vi "Sweep Pattern Dialog.vi"(8 "error in (no error)":errorcluster, 11 "Sweep Settings In":T1 {"Sweep Max" format="%#_6p"; "Sweep Min" format="%#_6p"; "Sweep Type" items=["Single Point", "Sweep", "List"]}) -> (0 "error out":errorcluster, 1 "Cancelled?":bool, 2 "Values":dbl[](array[numeric]), 3 "Sweep Settings Out":T1={"Sweep Type"=0, "Quantity"=enum."Undefined", "Base Unit"=enum."No", "Convention Unit"=enum."No", "Sweep Min"=0.0, "Sweep Max"=0.0, "Sweep NrOfPts"=0, "Values"=[0.0]} {"Sweep Max" format="%#_6p"; "Sweep Min" format="%#_6p"; "Sweep Type" items=["Single Point", "Sweep", "List"]})   [LabVIEW 2023, in "NI_HFNetworkAnalysis.lvlib"]
doc: "Dialog box allowing one to define a sweep pattern for double-precision floating point values."
uses:
  NI_HFNetworkAnalysis.lvlib
  Controls/SweepSettings.ctl
  Controls/Quantity.ctl
  Controls/Unit.ctl
  <vilib>/Utility/miscctls.llb/LVRowAndColumnTypeDef.ctl
  Support VIs/Convert Unit (DBL).vi
  Support VIs/Convert Unit (DBL Array).vi
panel:
  in  "Panel":enum32{"Page 1", "Page 3"}(tab)
  in  "Sweep Settings":T4 caption="Single" {"value3" format="%#_6p"; "value2" format="%#_6p"; "value1" format="%#_6p"}
  in  "Custom Value":T5 {"value1" format="%#_6p"}
  out "Custom List":string[][](table)
  in  "Cancel Button":bool
  in  "OK Button":bool
  in  "Type":u16(ring) caption="Type:" items=["Single Point", "Sweep", "List"]
  in  "Unit":u16(ring) caption="Unit:" items=["No"=0, "dB"=7]
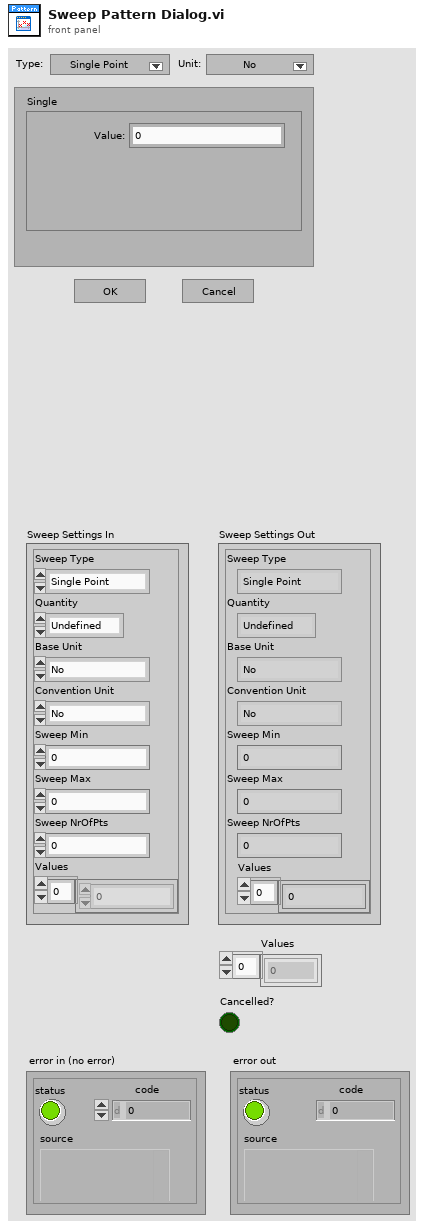
[diagram p1: front panel]
types:
  T1 = typedef "NI_HFNetworkAnalysis.lvlib/SweepSettings.ctl" = cluster{"Sweep Type":u16, "Quantity":T2, "Base Unit":T3, "Convention Unit":T3, "Sweep Min":dbl, "Sweep Max":dbl, "Sweep NrOfPts":u32, "Values":dbl[]}
  T2 = typedef "NI_HFNetworkAnalysis.lvlib/Quantity.ctl" = enum16{"Undefined", "V", "I", "A", "B", "P", "Z", "PowerRatio", "Gamma", "Index"}
  T3 = typedef "NI_HFNetworkAnalysis.lvlib/Unit.ctl" = enum16{"No", "s", "Hz", "V", "A", "Ohm", "W", "dB", "dBV", "dBA", "dBm", "percent", "rad", "deg"}
  T4 = cluster{"value1":dbl, "value2":dbl, "value3":dbl, "value4":u32, "MinMax":bool, "MinStep":bool}
  T5 = cluster{"value1":dbl, "Delete Point":bool, "Add Point":bool}
  T6 = typedef "LVRowAndColumnTypeDef.ctl" = cluster{"Row":i32, "Column":i32}
  T7 = enum8{"Enabled", "Disabled", "Disabled and Grayed Out"}
  T8 = cluster{"Sweep Type":u16, "Quantity":T2, "Base Unit":T3, "Convention Unit":u16, "Sweep Min":dbl, "Sweep Max":dbl, "Sweep NrOfPts":u32, "Values":dbl[]}
  T9 = cluster{"Sweep Type":u16, "Quantity":T2, "Base Unit":T3, "Convention Unit":u16, "regularSweepMin":dbl, "regularSweepMax":dbl, "regularSweepNrOfPts":u32, "Values":dbl[]}
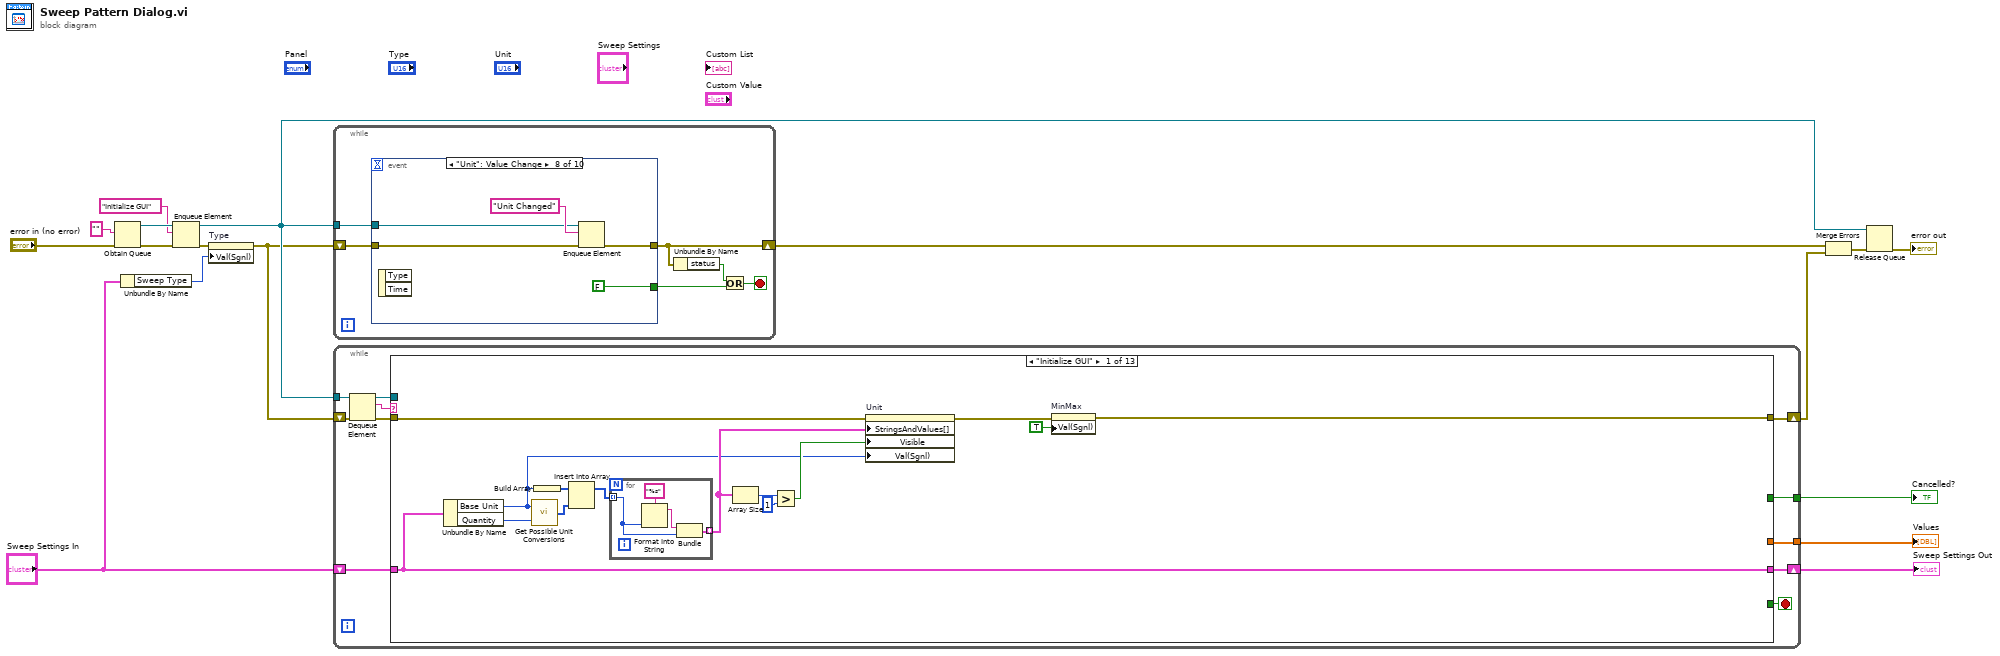
[diagram p0: block diagram]
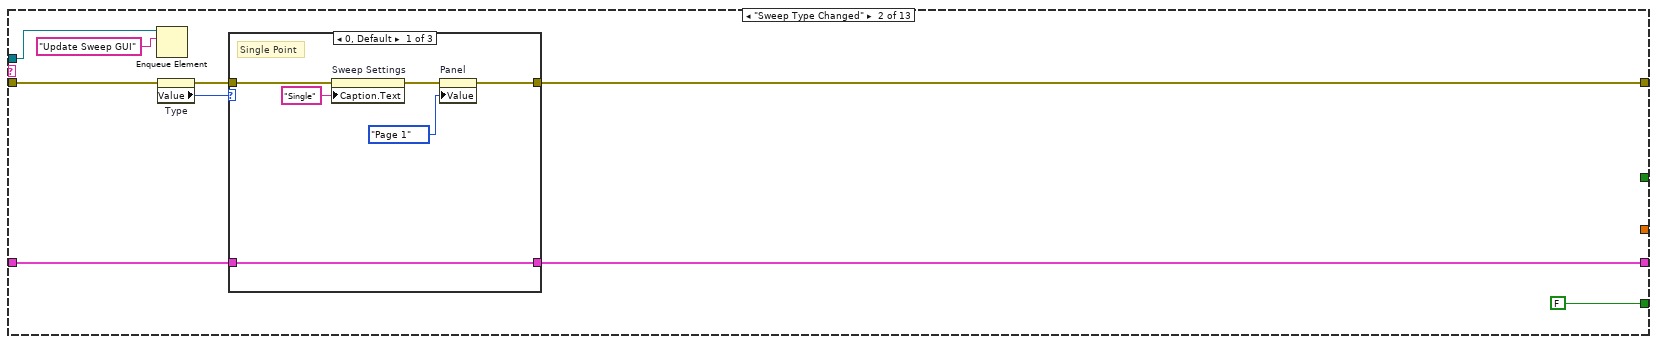
[diagram p2: hidden frame]
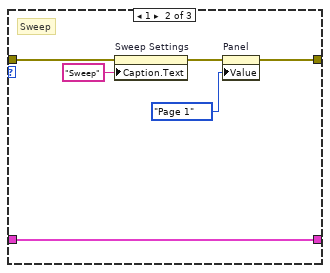
[diagram p3: hidden frame]
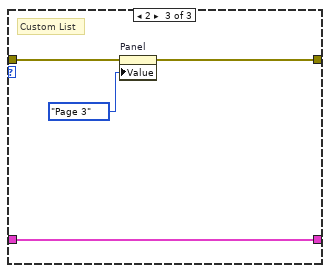
[diagram p4: hidden frame]
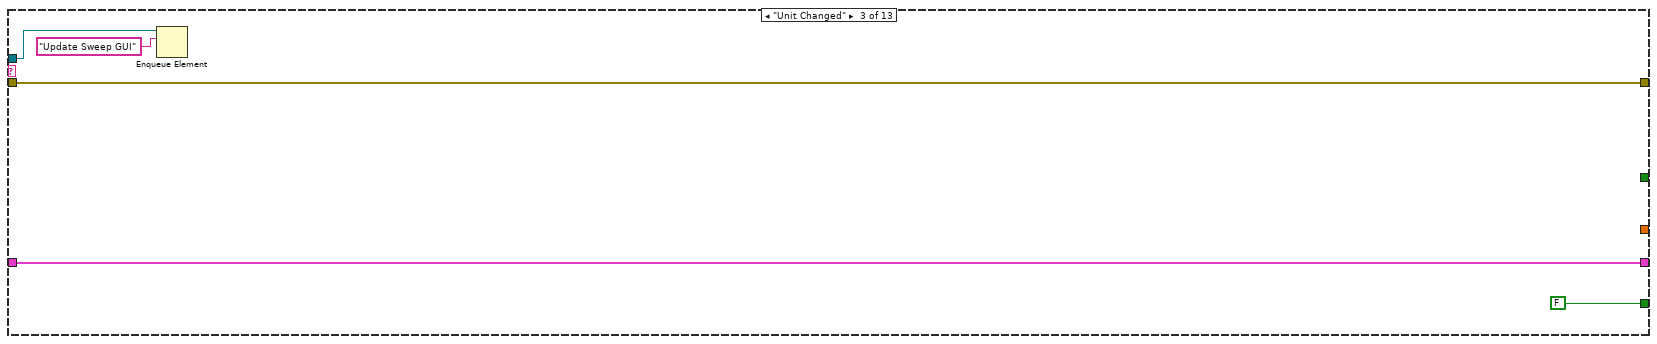
[diagram p5: hidden frame]
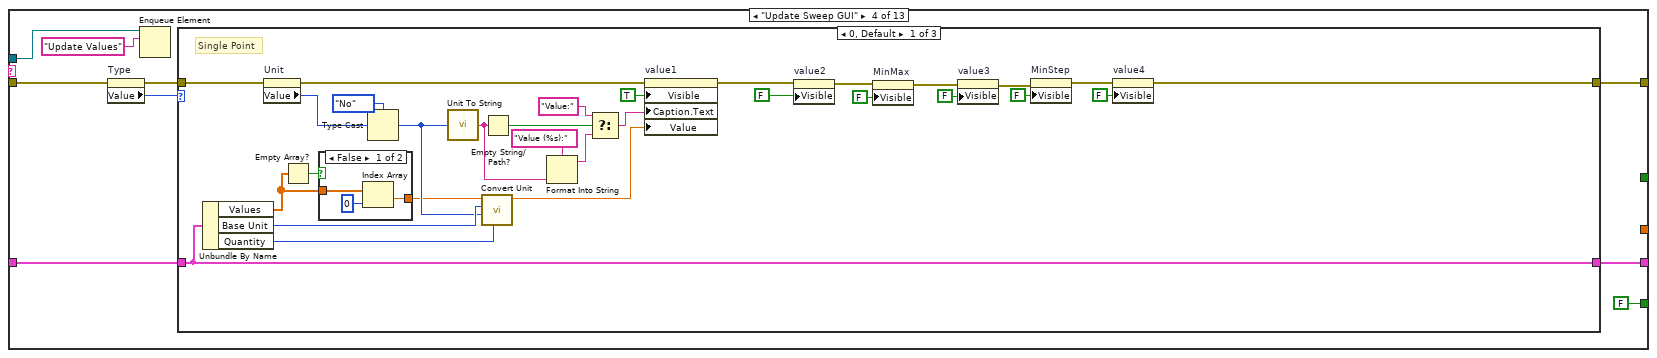
[diagram p6: hidden frame]
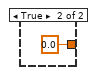
[diagram p7: hidden frame]
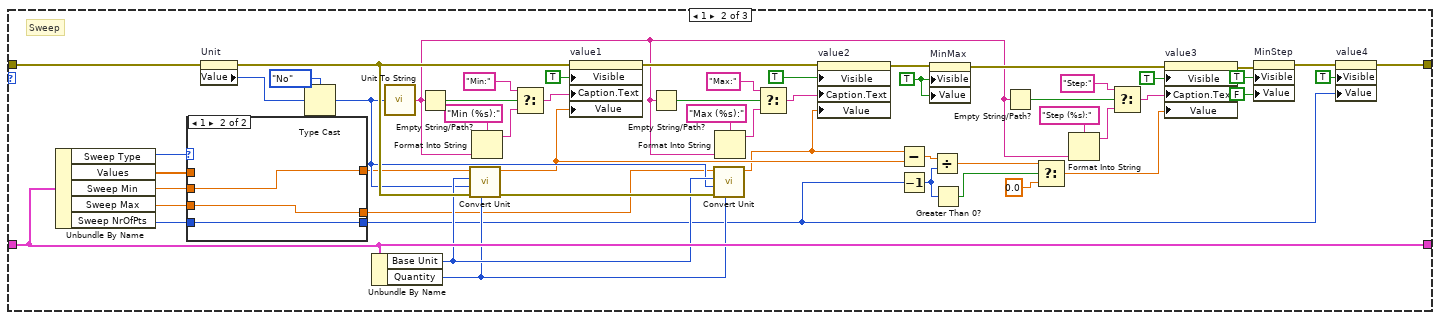
[diagram p8: hidden frame]
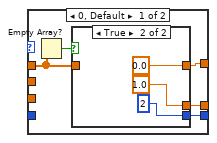
[diagram p9: hidden frame]
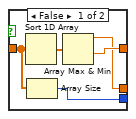
[diagram p10: hidden frame]
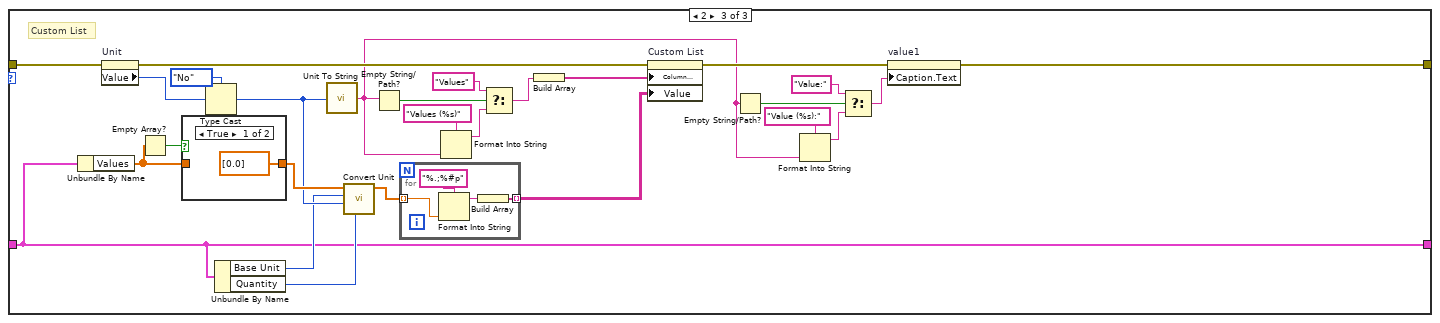
[diagram p11: hidden frame]
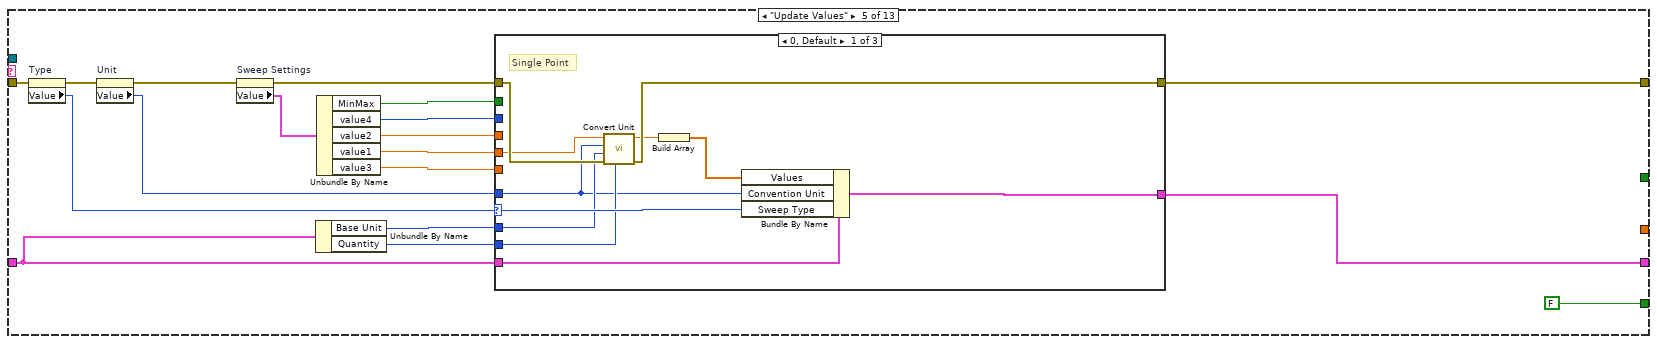
[diagram p13: hidden frame]
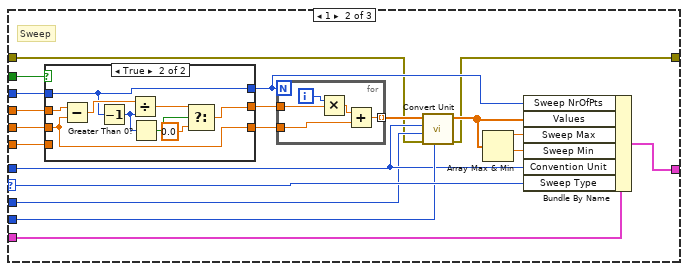
[diagram p14: hidden frame]
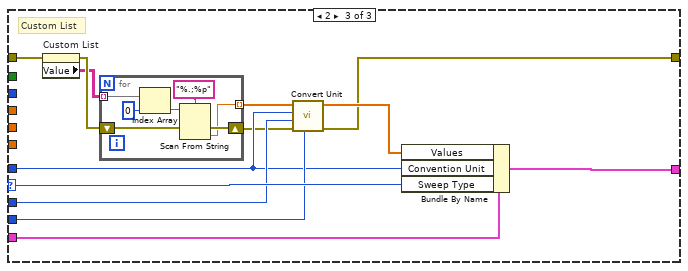
[diagram p16: hidden frame]
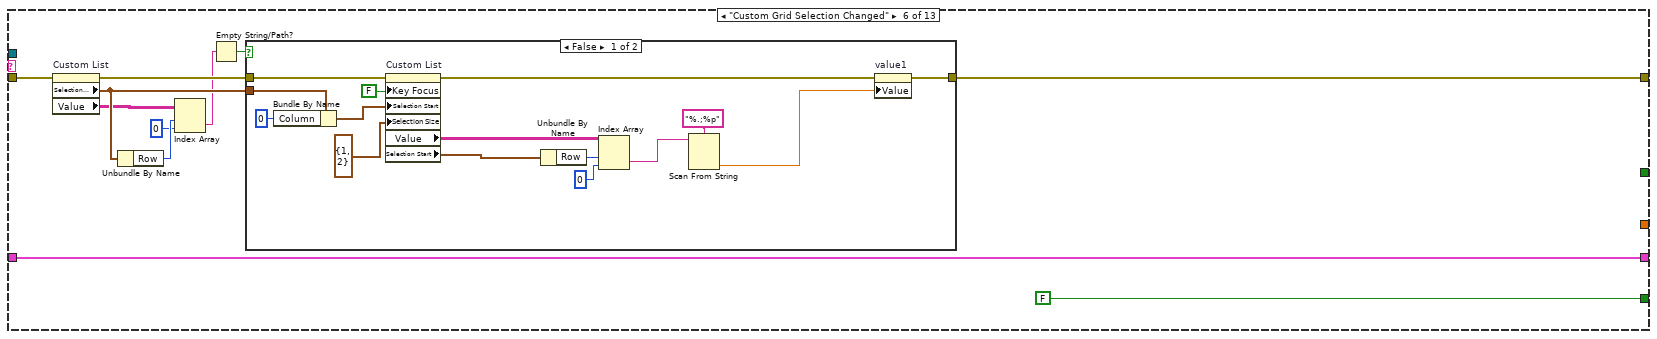
[diagram p17: hidden frame]
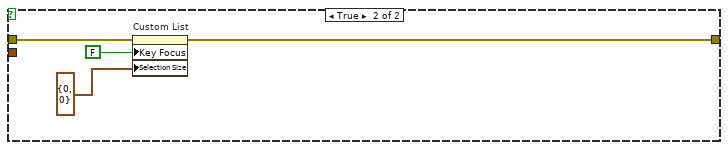
[diagram p18: hidden frame]
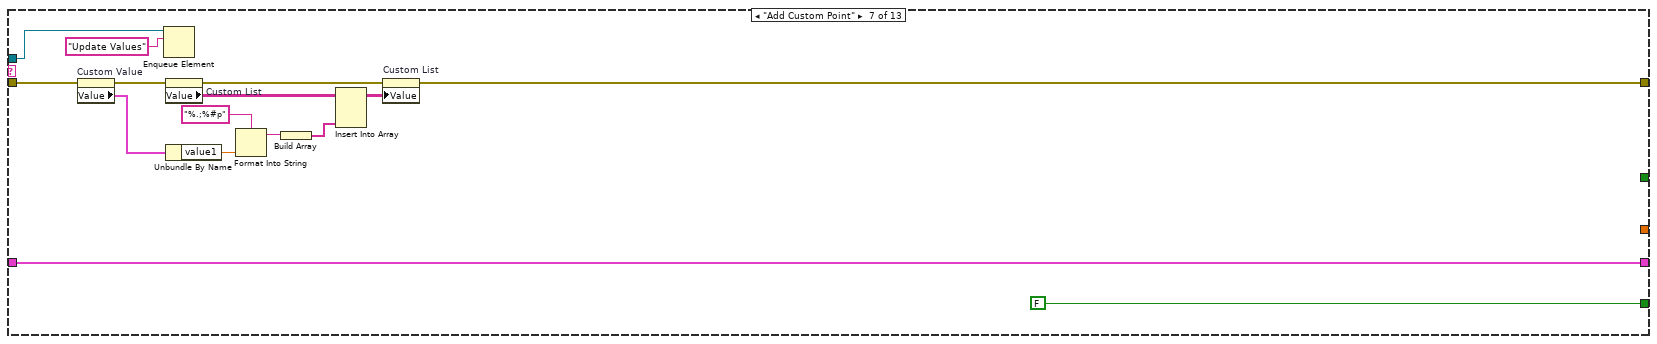
[diagram p19: hidden frame]
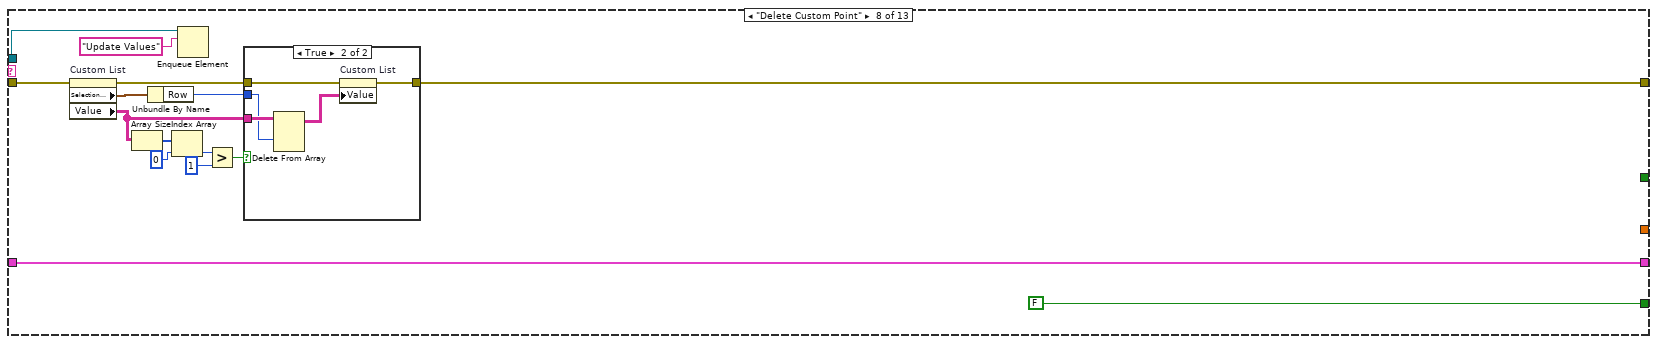
[diagram p20: hidden frame]
diagram:
  n1 = Obtain Queue(element data type="", error in (no error)="error in (no error)") -> (queue out=w13:refnum<queue>, error out=w7:errorcluster)  [unwired: 3 in, 1 out]
  n2 = Unbundle By Name("Sweep Settings In") -> ("Sweep Type"=w2:u16)
  n3 = Enqueue Element(queue=w13, element="Initialize GUI", error in (no error)=w7) -> (queue out=w8:refnum<queue>, error out=w6:errorcluster)  [unwired: 1 in, 1 out]
  n4 = property on="Type" class="Ring (strict)"(error in=w6, "Val(Sgnl)"=w2) -> (error out=w5:errorcluster)  [unwired: 1 in, 1 out]
  n5 = while {
    shift-right: [w18] -> w16
    shift-left: w5 -> [w20]
    tunnel: w8 -> [w19]
    stop <- w23 stop-if-true
    n6 = event shown="[7] \"Unit\": Value Change" {
      selector: _ -> [_ _ _ _ _ _ _ _ _ _]
      dyn-events: _ -> [_ _ _ _ _ _ _ _ _ _]
      timeout: _ -> [_ _ _ _ _ _ _ _ _ _]
      tunnel: [FALSE FALSE FALSE _ _ FALSE FALSE FALSE TRUE TRUE] -> w21
      tunnel: w20 -> [w26 w31 w36 w41 w45 w47 w55 w65 w70 w75]
      tunnel: w19 -> [w24 w29 w34 w40 w44 w51 w59 w63 w68 w73]
      tunnel: [w27 w32 w37 w42 w46 w53 w61 w66 w71 w76] -> w18
      event "Type": Value Change {
        n7 = event-data() -> ()  [unwired: 1 in, 2 out]
        n8 = Enqueue Element(queue=w24, element="Sweep Type Changed", error in (no error)=w26) -> (error out=w27:errorcluster)  [unwired: 1 in, 2 out]
      }
      event "Custom List": Mouse Up {
        n9 = event-data() -> ()  [unwired: 1 in, 2 out]
        n10 = Enqueue Element(queue=w29, element="Custom Grid Selection Changed", error in (no error)=w31) -> (error out=w32:errorcluster)  [unwired: 1 in, 2 out]
      }
      event "Sweep Settings": Value Change {
        n11 = event-data() -> ()  [unwired: 1 in, 2 out]
        n12 = Enqueue Element(queue=w34, element="Sweep Settings Changed", error in (no error)=w36) -> (error out=w37:errorcluster)  [unwired: 1 in, 2 out]
      }
      event "Sweep Settings.MinMax": Value Change {
        n13 = event-data() -> ()  [unwired: 1 in, 2 out]
        n14 = Enqueue Element(queue=w40, element="Max Selection Changed", error in (no error)=w41) -> (error out=w42:errorcluster)  [unwired: 1 in, 2 out]
      }
      event "Sweep Settings.MinStep": Value Change {
        n15 = event-data() -> ()  [unwired: 1 in, 2 out]
        n16 = Enqueue Element(queue=w44, element="Step Selection Changed", error in (no error)=w45) -> (error out=w46:errorcluster)  [unwired: 1 in, 2 out]
      }
      event "Custom Value.Add Point": Value Change {
        # "Reset Button"
        n17 = event-data() -> ("CtlRef"=w50:refnum<vi>, "OldVal"=w49:bool)  [unwired: 1 in]
        n18 = property class="Bool (strict)"(reference=w50, error in=w47, "Value"=w49) -> (error out=w48:errorcluster)  [unwired: 1 out]
        n19 = Enqueue Element(queue=w51, element="Add Custom Point", error in (no error)=w48) -> (error out=w53:errorcluster)  [unwired: 1 in, 2 out]
      }
      event "Custom Value.Delete Point": Value Change {
        # "Reset Button"
        n20 = event-data() -> ("CtlRef"=w58:refnum<vi>, "OldVal"=w57:bool)  [unwired: 1 in]
        n21 = property class="Bool (strict)"(reference=w58, error in=w55, "Value"=w57) -> (error out=w56:errorcluster)  [unwired: 1 out]
        n22 = Enqueue Element(queue=w59, element="Delete Custom Point", error in (no error)=w56) -> (error out=w61:errorcluster)  [unwired: 1 in, 2 out]
      }
      event "Unit": Value Change {
        n23 = event-data() -> ()  [unwired: 1 in, 2 out]
        n24 = Enqueue Element(queue=w63, element="Unit Changed", error in (no error)=w65) -> (error out=w66:errorcluster)  [unwired: 1 in, 2 out]
      }
      event "Cancel Button": Value Change {
        n25 = event-data() -> ()  [unwired: 1 in, 2 out]
        n26 = Enqueue Element(queue=w68, element="Cancel", error in (no error)=w70) -> (error out=w71:errorcluster)  [unwired: 1 in, 2 out]
      }
      event "OK Button": Value Change {
        n27 = event-data() -> ()  [unwired: 1 in, 2 out]
        n28 = Enqueue Element(queue=w73, element="OK", error in (no error)=w75) -> (error out=w76:errorcluster)  [unwired: 1 in, 2 out]
      }
    }
    n29 = Unbundle By Name(w18) -> ("status"=w22:bool)
    n30 = Or(x=w22, y=w21) -> (x .or. y?=w23:bool)
  }
  n31 = while {
    tunnel: w8 -> [w88]
    shift-right: [w84] -> w15
    shift-left: w5 -> [w87]
    tunnel: [w81] -> w12
    shift-right: [w79] -> w1
    shift-left: "Sweep Settings In" -> [w80]
    tunnel: [w78] -> w10
    stop <- w82 stop-if-true
    n32 = Dequeue Element(queue=w88, error in (no error)=w87) -> (queue out=w85:refnum<queue>, element=w83:string, error out=w86:errorcluster)  [unwired: 1 in, 1 out]
    n33 = case shown="\"Initialize GUI\"" w83 {
      tunnel: w86 -> [w96 w115 w136 w143 w300 w379 w403 w428 w446 w476 w479 w491 w496]
      tunnel: w85 -> [_ w110 w134 w144 _ _ w408 w416 w448 _ _ _ _]
      tunnel: [w89 w112 w136 w140 w299 w377 w411 w418 w435 w477 w488 w491 w494] -> w84
      tunnel: [_ FALSE FALSE FALSE FALSE FALSE FALSE FALSE FALSE _ _ TRUE TRUE] -> w82
      tunnel: [_ _ _ _ _ _ _ _ _ _ _ TRUE FALSE] -> w81
      tunnel: w80 -> [w92 w108 w132 w138 w286 w369 w405 w414 w447 w467 w478 _ w495]
      tunnel: [w92 w107 w132 w137 w289 w369 w405 w414 w447 w467 w478 w489 w495] -> w79
      tunnel: [_ _ _ _ _ _ _ _ _ _ _ _ w501] -> w78
      frame "Initialize GUI" {
        n34 = Unbundle By Name(w92) -> ("Base Unit"=w93:T3, "Quantity"=w102:T2)
        n35 = call "Get Possible Unit Conversions.vi"("Quantity"=w102, "Base Unit"=w93) -> ("Possible Target Units"=w100:T3[])
        n36 = Build Array(w93) -> (w101:T3[])
        n37 = Insert Into Array(array=w101, new element=w100) -> (w99:T3[])  [unwired: 1 in]
        n38 = for {
          tunnel: w99 -> [w104] mode=indexing
          tunnel: [w103] -> w95 mode=indexing
          n39 = Format Into String(format string="%s", w104) -> (resulting string=w105:string)  [unwired: 2 in, 1 out]
          n40 = Bundle(w105, "Base Unit"=w104) -> (w103:cluster{string, "Base Unit":T3})  [unwired: 1 in]
        }
        n41 = Array Size(array=w95) -> (size(s)=w98:i32)
        n42 = Greater?(x=w98, y=1) -> (0:w94:bool)
        n43 = property on="Unit" class="Ring (strict)"(error in=w96, "StringsAndValues[]"=w95, "Visible"=w94, "Val(Sgnl)"=w93) -> (error out=w91:errorcluster)  [unwired: 1 in, 1 out]
        n44 = property on="MinMax" class="Bool (strict)"(error in=w91, "Val(Sgnl)"=TRUE ("Value (Signaling)")) -> (error out=w89:errorcluster)  [unwired: 1 in, 1 out]
      }
      frame "Sweep Type Changed" {
        n45 = Enqueue Element(queue=w110, element="Update Sweep GUI") -> ()  [unwired: 2 in, 3 out]
        n46 = property on="Type" class="Ring (strict)"(error in=w115) -> (error out=w113:errorcluster, "Value"=w114:u16)  [unwired: 1 in, 1 out]
        n47 = case shown="0, Default" w114 {
          tunnel: w113 -> [w118 w124 w128]
          tunnel: [w120 w126 w130] -> w112
          tunnel: w108 -> [w119 w125 w129]
          tunnel: [w119 w125 w129] -> w107
          frame 0, Default {
            # "Single Point"
            n48 = property on="Sweep Settings" class="Clust (strict)"(error in=w118, "Caption.Text"="Single") -> (error out=w117:errorcluster)  [unwired: 1 in, 1 out]
            n49 = property on="Panel" class="TabCtl (strict)"(error in=w117, "Value"=enum32{"Page 1", "Page 3"}."Page 1" ("LeftPanel")) -> (error out=w120:errorcluster)  [unwired: 1 in, 1 out]
          }
          frame 1 {
            # "Sweep"
            n50 = property on="Sweep Settings" class="Clust (strict)"(error in=w124, "Caption.Text"="Sweep") -> (error out=w123:errorcluster)  [unwired: 1 in, 1 out]
            n51 = property on="Panel" class="TabCtl (strict)"(error in=w123, "Value"=enum32{"Page 1", "Page 3"}."Page 1" ("LeftPanel")) -> (error out=w126:errorcluster)  [unwired: 1 in, 1 out]
          }
          frame 2 {
            # "Custom List"
            n52 = property on="Panel" class="TabCtl (strict)"(error in=w128, "Value"=enum32{"Page 1", "Page 3"}."Page 3" ("LeftPanel")) -> (error out=w130:errorcluster)  [unwired: 1 in, 1 out]
          }
        }
      }
      frame "Unit Changed" {
        n53 = Enqueue Element(queue=w134, element="Update Sweep GUI") -> ()  [unwired: 2 in, 3 out]
      }
      frame "Update Sweep GUI" {
        n54 = property on="Type" class="Ring (strict)"(error in=w143) -> (error out=w141:errorcluster, "Value"=w142:u16)  [unwired: 1 in, 1 out]
        n55 = Enqueue Element(queue=w144, element="Update Values") -> ()  [unwired: 2 in, 3 out]
        n56 = case shown="0, Default" w142 {
          tunnel: w141 -> [w170 w226 w271]
          tunnel: [w148 w200 w269] -> w140
          tunnel: w138 -> [w168 w208 w251]
          tunnel: [w168 w208 w251] -> w137
          frame 0, Default {
            # "Single Point"
            n57 = Unbundle By Name(w168) -> ("Values"=w161:dbl[], "Base Unit"=w151:T3, "Quantity"=w149:T2)
            n58 = property on="Unit" class="Ring (strict)"(error in=w170) -> (error out=w169:errorcluster, "Value"=w158:u16)  [unwired: 1 in, 1 out]
            n59 = Empty Array?(array=w161) -> (empty?=w160:bool)
            n60 = case shown="False" w160 {
              tunnel: w161 -> [w178 _]
              tunnel: [w176 0.0] -> w147
              frame False {
                n61 = Index Array(array=w178, index=0) -> (element=w176:dbl)
              }
              frame True {
              }
            }
            n62 = Type Cast(type=Unit."No" ("Unit"), x=w158) -> (*(type *) &x=w150:T3)
            n63 = call "Unit To String.vi"("Unit"=w150) -> ("String"=w153:string)
            n64 = call-poly "Convert Unit.vi"("Quantity"=w149, "Target Unit"=w150, "Base Unit"=w151, "Data"=w147) -> ("Converted Data"=w146:dbl)  [unwired: 3 in, 1 out]
            n65 = Empty String/Path?(string/path=w153) -> (empty?=w157:bool)
            n66 = Format Into String(format string="Value (%s):", w153) -> (resulting string=w155:string)  [unwired: 2 in, 1 out]
            n67 = Select(t="Value:", s=w157, f=w155) -> (s? t:f=w152:string)
            n68 = property on="value1" class="DigNum (strict)"(error in=w169, "Visible"=TRUE, "Caption.Text"=w152, "Value"=w146) -> (error out=w173:errorcluster)  [unwired: 1 in, 1 out]
            n69 = property on="value2" class="DigNum (strict)"(error in=w173, "Visible"=FALSE) -> (error out=w166:errorcluster)  [unwired: 1 in, 1 out]
            n70 = property on="MinMax" class="Bool (strict)"(error in=w166, "Visible"=FALSE) -> (error out=w165:errorcluster)  [unwired: 1 in, 1 out]
            n71 = property on="value3" class="DigNum (strict)"(error in=w165, "Visible"=FALSE) -> (error out=w163:errorcluster)  [unwired: 1 in, 1 out]
            n72 = property on="MinStep" class="Bool (strict)"(error in=w163, "Visible"=FALSE) -> (error out=w162:errorcluster)  [unwired: 1 in, 1 out]
            n73 = property on="value4" class="DigNum (strict)"(error in=w162, "Visible"=FALSE) -> (error out=w148:errorcluster)  [unwired: 1 in, 1 out]
          }
          frame 1 {
            w197 = TRUE ("Visible")
            # "Sweep"
            n74 = Unbundle By Name(w208) -> ("Sweep Type"=w207:u16, "Values"=w206:dbl[], "Sweep Min"=w205:dbl, "Sweep Max"=w204:dbl, "Sweep NrOfPts"=w203:u32)
            n75 = case shown="1" w207 {
              tunnel: [w236 w249] -> w183
              tunnel: w206 -> [w237 _]
              tunnel: w205 -> [_ w249]
              tunnel: w204 -> [_ w248]
              tunnel: w203 -> [_ w247]
              tunnel: [w235 w248] -> w181
              tunnel: [w234 w247] -> w198
              frame 0, Default {
                n76 = Empty Array?(array=w237) -> (empty?=w238:bool)
                n77 = case shown="True" w238 {
                  tunnel: w237 -> [w240 _]
                  tunnel: [w242 0.0] -> w236
                  tunnel: [w241 1.0] -> w235
                  tunnel: [w239 u32 2 ("regularSweepNrOfPts")] -> w234
                  frame False {
                    n78 = Sort 1D Array(array=w240) -> (sorted array=w243:dbl[])
                    n79 = Array Size(array=w240) -> (size(s)=w239:i32)
                    n80 = Array Max & Min(array=w243) -> (max value=w241:dbl, min value=w242:dbl)  [unwired: 2 out]
                  }
                  frame True {
                  }
                }
              }
              frame 1 {
              }
            }
            n81 = property on="Unit" class="Ring (strict)"(error in=w226) -> (error out=w232:errorcluster, "Value"=w219:u16)  [unwired: 1 in, 1 out]
            n82 = Type Cast(type=Unit."No" ("Unit"), x=w219) -> (*(type *) &x=w195:T3)
            n83 = Unbundle By Name(w208) -> ("Base Unit"=w202:T3, "Quantity"=w201:T2)
            n84 = call "Unit To String.vi"("Unit"=w195) -> ("String"=w186:string)
            n85 = Empty String/Path?(string/path=w186) -> (empty?=w218:bool)
            n86 = call-poly "Convert Unit.vi"("Quantity"=w201, "error in (no error)"=w232, "Target Unit"=w195, "Base Unit"=w202, "Data"=w183) -> ("error out"=w233:errorcluster, "Converted Data"=w182:dbl)  [unwired: 2 in]
            n87 = Format Into String(format string="Min (%s):", w186) -> (resulting string=w216:string)  [unwired: 2 in, 1 out]
            n88 = Select(t="Min:", s=w218, f=w216) -> (s? t:f=w214:string)
            n89 = property on="value1" class="DigNum (strict)"(error in=w232, "Visible"=TRUE, "Caption.Text"=w214, "Value"=w182) -> (error out=w229:errorcluster)  [unwired: 1 in, 1 out]
            n90 = Empty String/Path?(string/path=w186) -> (empty?=w213:bool)
            n91 = call-poly "Convert Unit.vi"("Quantity"=w201, "error in (no error)"=w233, "Target Unit"=w195, "Base Unit"=w202, "Data"=w181) -> ("Converted Data"=w180:dbl)  [unwired: 2 in, 1 out]
            n92 = Format Into String(format string="Max (%s):", w186) -> (resulting string=w211:string)  [unwired: 2 in, 1 out]
            n93 = Select(t="Max:", s=w213, f=w211) -> (s? t:f=w209:string)
            n94 = property on="value2" class="DigNum (strict)"(error in=w229, "Visible"=TRUE, "Caption.Text"=w209, "Value"=w180) -> (error out=w225:errorcluster)  [unwired: 1 in, 1 out]
            n95 = Subtract(x=w180, y=w182) -> (x-y=w199:dbl)
            n96 = Decrement(x=w198) -> (x-1=w193:u32)
            n97 = property on="MinMax" class="Bool (strict)"(error in=w225, "Visible"=w197, "Value"=w197) -> (error out=w224:errorcluster)  [unwired: 1 in, 1 out]
            n98 = Divide(x=w199, y=w193) -> (x/y=w192:dbl)
            n99 = Greater Than 0?(x=w193) -> (x > 0?=w194:bool)
            n100 = Empty String/Path?(string/path=w186) -> (empty?=w190:bool)
            n101 = Select(t=w192, s=w194, f=0.0) -> (s? t:f=w185:dbl)
            n102 = Format Into String(format string="Step (%s):", w186) -> (resulting string=w188:string)  [unwired: 2 in, 1 out]
            n103 = Select(t="Step:", s=w190, f=w188) -> (s? t:f=w184:string)
            n104 = property on="value3" class="DigNum (strict)"(error in=w224, "Visible"=TRUE, "Caption.Text"=w184, "Value"=w185) -> (error out=w222:errorcluster)  [unwired: 1 in, 1 out]
            n105 = property on="MinStep" class="Bool (strict)"(error in=w222, "Visible"=TRUE, "Value"=FALSE) -> (error out=w221:errorcluster)  [unwired: 1 in, 1 out]
            n106 = property on="value4" class="DigNum (strict)"(error in=w221, "Visible"=TRUE, "Value"=w198) -> (error out=w200:errorcluster)  [unwired: 1 in, 1 out]
          }
          frame 2 {
            # "Custom List"
            n107 = Unbundle By Name(w251) -> ("Values"=w274:dbl[])
            n108 = property on="Unit" class="Ring (strict)"(error in=w271) -> (error out=w270:errorcluster, "Value"=w272:u16)  [unwired: 1 in, 1 out]
            n109 = Empty Array?(array=w274) -> (empty?=w276:bool)
            n110 = case shown="True" w276 {
              tunnel: [dbl[] [0.0] w282] -> w255
              tunnel: w274 -> [_ w282]
              frame True {
              }
              frame False {
              }
            }
            n111 = Type Cast(type=Unit."No" ("Unit"), x=w272) -> (*(type *) &x=w254:T3)
            n112 = Unbundle By Name(w251) -> ("Base Unit"=w253:T3, "Quantity"=w252:T2)
            n113 = call "Unit To String.vi"("Unit"=w254) -> ("String"=w257:string)
            n114 = call-poly "Convert Unit.vi"("Quantity"=w252, "Target Unit"=w254, "Base Unit"=w253, "Data"=w255) -> ("Converted Data"=w250:dbl[])  [unwired: 3 in, 1 out]
            n115 = Empty String/Path?(string/path=w257) -> (empty?=w268:bool)
            n116 = for {
              tunnel: [w280] -> w256 mode=indexing
              tunnel: w250 -> [w277] mode=indexing
              n117 = Format Into String(format string="%.;%#p", w277) -> (resulting string=w278:string)  [unwired: 2 in, 1 out]
              n118 = Build Array(w278) -> (w280:string[])
            }
            n119 = Format Into String(format string="Values (%s)", w257) -> (resulting string=w267:string)  [unwired: 2 in, 1 out]
            n120 = Select(t="Values", s=w268, f=w267) -> (s? t:f=w264:string)
            n121 = Build Array(w264) -> (w263:string[])
            n122 = property on="Custom List" class="Tbl (strict)"(error in=w270, "Column Headers[]"=w263, "Value"=w256) -> (error out=w275:errorcluster)  [unwired: 1 in, 1 out]
            n123 = Empty String/Path?(string/path=w257) -> (empty?=w262:bool)
            n124 = Format Into String(format string="Value (%s):", w257) -> (resulting string=w261:string)  [unwired: 2 in, 1 out]
            n125 = Select(t="Value:", s=w262, f=w261) -> (s? t:f=w259:string)
            n126 = property on="value1" class="DigNum (strict)"(error in=w275, "Caption.Text"=w259) -> (error out=w269:errorcluster)  [unwired: 1 in, 1 out]
          }
        }
      }
      frame "Update Values" {
        n127 = property on="Type" class="Ring (strict)"(error in=w300) -> (error out=w297:errorcluster, "Value"=w294:u16)  [unwired: 1 in, 1 out]
        n128 = property on="Unit" class="Ring (strict)"(error in=w297) -> (error out=w288:errorcluster, "Value"=w296:u16)  [unwired: 1 in, 1 out]
        n129 = property on="Sweep Settings" class="Clust (strict)"(error in=w288) -> (error out=w287:errorcluster, "Value"=w295:T4)  [unwired: 1 in, 1 out]
        n130 = Unbundle By Name(w286) -> ("Base Unit"=w285:T3, "Quantity"=w284:T2)
        n131 = Unbundle By Name(w295) -> ("MinMax"=w283:bool, "value4"=w290:u32, "value2"=w291:dbl, "value1"=w292:dbl, "value3"=w293:dbl)
        n132 = case shown="0, Default" w294 {
          selector: w294 -> [w309 w330 w359]
          tunnel: [w311 w313 w350] -> w299
          tunnel: [w308 w331 w358] -> w289
          tunnel: w296 -> [w304 w317 w352]
          tunnel: w293 -> [_ w323 _]
          tunnel: w292 -> [w302 w325 _]
          tunnel: w291 -> [_ w328 _]
          tunnel: w290 -> [_ w327 _]
          tunnel: w287 -> [w310 w312 w357]
          tunnel: w286 -> [w307 w329 w356]
          tunnel: w285 -> [w306 w316 w353]
          tunnel: w284 -> [w305 w318 w354]
          tunnel: w283 -> [_ w322 _]
          frame 0, Default {
            # "Single Point"
            n133 = call-poly "Convert Unit.vi"("Quantity"=w305, "error in (no error)"=w310, "Target Unit"=w306, "Base Unit"=w304, "Data"=w302) -> ("error out"=w311:errorcluster, "Converted Data"=w303:dbl)  [unwired: 2 in]
            n134 = Build Array(w303) -> (w301:dbl[])
            n135 = Bundle By Name(cluster=w307, "Values"=w301, "Convention Unit"=w304, "Sweep Type"=w309) -> (w308:T8)
          }
          frame 1 {
            # "Sweep"
            n136 = case shown="True" w322 {
              tunnel: w328 -> [_ w343]
              tunnel: w327 -> [w332 w340]
              tunnel: [w333 w335] -> w326
              tunnel: w325 -> [w334 w341]
              tunnel: [w334 w341] -> w324
              tunnel: w323 -> [w333 _]
              tunnel: [w332 w340] -> w319
              frame False {
              }
              frame True {
                n137 = Subtract(x=w343, y=w341) -> (x-y=w342:dbl)
                n138 = Decrement(x=w340) -> (x-1=w339:u32)
                n139 = Divide(x=w342, y=w339) -> (x/y=w336:dbl)
                n140 = Greater Than 0?(x=w339) -> (x > 0?=w338:bool)
                n141 = Select(t=w336, s=w338, f=0.0) -> (s? t:f=w335:dbl)
              }
            }
            n142 = for {
              N: w319 -> [_]
              tunnel: w326 -> [w348]
              tunnel: w324 -> [w345]
              tunnel: [w344] -> w315 mode=indexing
              i -> [w347]
              n143 = Multiply(x=w347, y=w348) -> (x*y=w346:dbl)
              n144 = Add(x=w346, y=w345) -> (x+y=w344:dbl)
            }
            n145 = call-poly "Convert Unit.vi"("Quantity"=w318, "error in (no error)"=w312, "Target Unit"=w316, "Base Unit"=w317, "Data"=w315) -> ("error out"=w313:errorcluster, "Converted Data"=w314:dbl[])  [unwired: 2 in]
            n146 = Array Max & Min(array=w314) -> (max value=w321:dbl, min value=w320:dbl)  [unwired: 2 out]
            n147 = Bundle By Name(cluster=w329, "Sweep NrOfPts"=w319, "Values"=w314, "Sweep Max"=w321, "Sweep Min"=w320, "Convention Unit"=w317, "Sweep Type"=w330) -> (w331:T8)
          }
          frame 2 {
            # "Custom List"
            n148 = property on="Custom List" class="Tbl (strict)"(error in=w357) -> (error out=w361:errorcluster, "Value"=w360:string[][])  [unwired: 1 in, 1 out]
            n149 = for {
              tunnel: w360 -> [w365] mode=indexing
              tunnel: [w362] -> w355 mode=indexing
              shift-right: [w363] -> w349
              shift-left: w361 -> [w364]
              n150 = Index Array(array=w365, index=0 ("disabled index (col)")) -> (element=w368:string)
              n151 = Scan From String(format string="%.;%p", input string=w368, error in=w364) -> (error out=w363:errorcluster, output 1=w362:dbl)  [unwired: 2 in, 2 out]
            }
            n152 = call-poly "Convert Unit.vi"("Quantity"=w354, "error in (no error)"=w349, "Target Unit"=w353, "Base Unit"=w352, "Data"=w355) -> ("error out"=w350:errorcluster, "Converted Data"=w351:dbl[])  [unwired: 2 in]
            n153 = Bundle By Name(cluster=w356, "Values"=w351, "Convention Unit"=w352, "Sweep Type"=w359) -> (w358:T8)
          }
        }
      }
      frame "Custom Grid Selection Changed" {
        n154 = property on="Custom List" class="Tbl (strict)"(error in=w379) -> (error out=w378:errorcluster, "Selection Start"=w376:T6, "Value"=w375:string[][])  [unwired: 1 in, 1 out]
        n155 = Unbundle By Name(w376) -> ("Row"=w374:i32)
        n156 = Index Array(array=w375, index (row)=w374, index (col)=0 ("disabled index (col)")) -> (element=w371:string)
        n157 = Empty String/Path?(string/path=w371) -> (empty?=w372:bool)
        n158 = case shown="False" w372 {
          tunnel: w376 -> [w392 _]
          tunnel: w378 -> [w389 w398]
          tunnel: [w382 w397] -> w377
          frame False {
            n159 = Bundle By Name(cluster=w392, "Column"=0) -> (w393:T6)
            n160 = property on="Custom List" class="Tbl (strict)"(error in=w389, "Key Focus"=FALSE, "Selection Start"=w393, "Selection Size"=T6 {"Row"=1, "Column"=2}) -> (error out=w381:errorcluster, "Value"=w386:string[][], "Selection Start"=w385:T6)  [unwired: 1 in, 1 out]
            n161 = Unbundle By Name(w385) -> ("Row"=w388:i32)
            n162 = Index Array(array=w386, index (row)=w388, index (col)=0 ("disabled index (col)")) -> (element=w384:string)
            n163 = Scan From String(format string="%.;%p", input string=w384) -> (output 1=w380:dbl)  [unwired: 3 in, 3 out]
            n164 = property on="value1" class="DigNum (strict)"(error in=w381, "Value"=w380) -> (error out=w382:errorcluster)  [unwired: 1 in, 1 out]
          }
          frame True {
            n165 = property on="Custom List" class="Tbl (strict)"(error in=w398, "Key Focus"=FALSE, "Selection Size"=T6 {"Row"=0, "Column"=0} ("Selection Start")) -> (error out=w397:errorcluster)  [unwired: 1 in, 1 out]
          }
        }
      }
      frame "Add Custom Point" {
        n166 = property on="Custom Value" class="Clust (strict)"(error in=w403) -> (error out=w402:errorcluster, "Value"=w413:T5)  [unwired: 1 in, 1 out]
        n167 = Enqueue Element(queue=w408, element="Update Values") -> ()  [unwired: 2 in, 3 out]
        n168 = property on="Custom List" class="Tbl (strict)"(error in=w402) -> (error out=w410:errorcluster, "Value"=w412:string[][])  [unwired: 1 in, 1 out]
        n169 = Unbundle By Name(w413) -> ("value1"=w404:dbl)
        n170 = Format Into String(format string="%.;%#p", w404) -> (resulting string=w401:string)  [unwired: 2 in, 1 out]
        n171 = Build Array(w401) -> (w400:string[])
        n172 = Insert Into Array(array=w412, new element=w400) -> (w409:string[][])  [unwired: 2 in]
        n173 = property on="Custom List" class="Tbl (strict)"(error in=w410, "Value"=w409) -> (error out=w411:errorcluster)  [unwired: 1 in, 1 out]
      }
      frame "Delete Custom Point" {
        n174 = property on="Custom List" class="Tbl (strict)"(error in=w428) -> (error out=w419:errorcluster, "Selection Start"=w421:T6, "Value"=w422:string[][])  [unwired: 1 in, 1 out]
        n175 = Array Size(array=w422) -> (size(s)=w427:i32[])
        n176 = Unbundle By Name(w421) -> ("Row"=w420:i32)
        n177 = Index Array(array=w427, index=0) -> (element=w425:i32)
        n178 = Enqueue Element(queue=w416, element="Update Values") -> ()  [unwired: 2 in, 3 out]
        n179 = Greater?(x=w425, y=1) -> (0:w423:bool)
        n180 = case shown="True" w423 {
          tunnel: w422 -> [_ w434]
          tunnel: w420 -> [_ w433]
          tunnel: w419 -> [w429 w432]
          tunnel: [w429 w431] -> w418
          frame False {
          }
          frame True {
            n181 = Delete From Array(array=w434, index (row)=w433) -> (array with subset deleted=w430:string[][])  [unwired: 2 in, 1 out]
            n182 = property on="Custom List" class="Tbl (strict)"(error in=w432, "Value"=w430) -> (error out=w431:errorcluster)  [unwired: 1 in, 1 out]
          }
        }
      }
      frame "Sweep Settings Changed" {
        n183 = property on="value1" class="DigNum (strict)"(error in=w446) -> (error out=w445:errorcluster, "Value"=w439:dbl)  [unwired: 1 in, 1 out]
        n184 = Enqueue Element(queue=w448, element="Update Values") -> ()  [unwired: 2 in, 3 out]
        n185 = property on="value2" class="DigNum (strict)"(error in=w445) -> (error out=w444:errorcluster, "Value"=w438:dbl)  [unwired: 1 in, 1 out]
        n186 = property on="value3" class="DigNum (strict)"(error in=w444) -> (error out=w443:errorcluster, "Value"=w437:dbl)  [unwired: 1 in, 1 out]
        n187 = property on="value4" class="DigNum (strict)"(error in=w443) -> (error out=w442:errorcluster, "Value"=w436:u32)  [unwired: 1 in, 1 out]
        n188 = property on="MinMax" class="Bool (strict)"(error in=w442) -> (error out=w441:errorcluster, "Value"=w440:bool)  [unwired: 1 in, 1 out]
        n189 = case shown="True" w440 {
          tunnel: w441 -> [w458 w466]
          tunnel: [w457 w465] -> w435
          tunnel: w439 -> [w452 w463]
          tunnel: w438 -> [_ w464]
          tunnel: w437 -> [w456 _]
          tunnel: w436 -> [w455 w462]
          frame False {
            n190 = Decrement(x=w455) -> (x-1=w454:u32)
            n191 = Multiply(x=w454, y=w456) -> (x*y=w453:dbl)
            n192 = Add(x=w453, y=w452) -> (x+y=w451:dbl)
            n193 = property on="value2" class="DigNum (strict)"(error in=w458, "Value"=w451) -> (error out=w457:errorcluster)  [unwired: 1 in, 1 out]
          }
          frame True {
            n194 = Subtract(x=w464, y=w463) -> (x-y=w460:dbl)
            n195 = Decrement(x=w462) -> (x-1=w461:u32)
            n196 = Divide(x=w460, y=w461) -> (x/y=w459:dbl)
            n197 = property on="value3" class="DigNum (strict)"(error in=w466, "Value"=w459) -> (error out=w465:errorcluster)  [unwired: 1 in, 1 out]
          }
        }
      }
      frame "Max Selection Changed" {
        n198 = property on="value2" class="DigNum (strict)"(error in=w476, "DisabledEnum"=T7."Enabled" ("Disabled")) -> (error out=w474:errorcluster)  [unwired: 1 in, 1 out]
        n199 = property on="value3" class="DigNum (strict)"(error in=w474, "DisabledEnum"=T7."Disabled and Grayed Out" ("Disabled")) -> (error out=w472:errorcluster)  [unwired: 1 in, 1 out]
        n200 = property on="MinMax" class="Bool (strict)"(error in=w472, "DisabledEnum"=T7."Disabled" ("Disabled")) -> (error out=w470:errorcluster)  [unwired: 1 in, 1 out]
        n201 = property on="MinStep" class="Bool (strict)"(error in=w470, "DisabledEnum"=T7."Enabled" ("Disabled"), "Value"=FALSE) -> (error out=w477:errorcluster)  [unwired: 1 in, 1 out]
      }
      frame "Step Selection Changed" {
        n202 = property on="value3" class="DigNum (strict)"(error in=w479, "DisabledEnum"=T7."Enabled" ("Disabled")) -> (error out=w486:errorcluster)  [unwired: 1 in, 1 out]
        n203 = property on="value2" class="DigNum (strict)"(error in=w486, "DisabledEnum"=T7."Disabled and Grayed Out" ("Disabled")) -> (error out=w484:errorcluster)  [unwired: 1 in, 1 out]
        n204 = property on="MinStep" class="Bool (strict)"(error in=w484, "DisabledEnum"=T7."Disabled" ("Disabled")) -> (error out=w482:errorcluster)  [unwired: 1 in, 1 out]
        n205 = property on="MinMax" class="Bool (strict)"(error in=w482, "DisabledEnum"=T7."Enabled" ("Disabled"), "Value"=FALSE) -> (error out=w488:errorcluster)  [unwired: 1 in, 1 out]
      }
      frame "Cancel", Default {
        w489 = T9 {"Sweep Type"=0, "Quantity"=enum."Undefined", "Base Unit"=enum."No", "Convention Unit"=0, "regularSweepMin"=0.0, "regularSweepMax"=0.0, "regularSweepNrOfPts"=0, "Values"=[0.0]}  # Sweep
        (unwired) cdb[] [] ("Values")
      }
      frame "OK" {
        n206 = Unbundle By Name(w495) -> ("Quantity"=w500:T2, "Values"=w499:dbl[], "Base Unit"=w498:T3, "Convention Unit"=w497:u16)
        n207 = call-poly "Convert Unit.vi"("Quantity"=w500, "error in (no error)"=w496, "Target Unit"=w497, "Base Unit"=w498, "Data"=w499) -> ("error out"=w493:errorcluster, "Converted Data"=w501:dbl[])  [unwired: 2 in]
        n208 = Merge Errors(w496, w493) -> (w494:errorcluster)
      }
    }
  }
  "Cancelled?" <- w12
  "Values" <- w10
  "Sweep Settings Out" <- w1
  n209 = Merge Errors(w16, w15) -> (w14:errorcluster)
  n210 = Release Queue(queue=w8, error in (no error)=w14) -> (error out=→"error out":errorcluster)  [unwired: 1 in, 2 out]
